vi "Find Config DB.vi"(8 "error in (no error)":errorcluster, 11 "Elevator Controller in":refnum<class "Elevator Controller.lvclass">) -> (0 "error out":errorcluster, 2 "DB Found?":bool, 3 "Elevator Controller out":refnum<class "Elevator Controller.lvclass">)   [LabVIEW 2019, in "Elevator Controller Actor.lvlib" / "Elevator Controller.lvclass"]
uses:
  Elevator Controller.lvclass
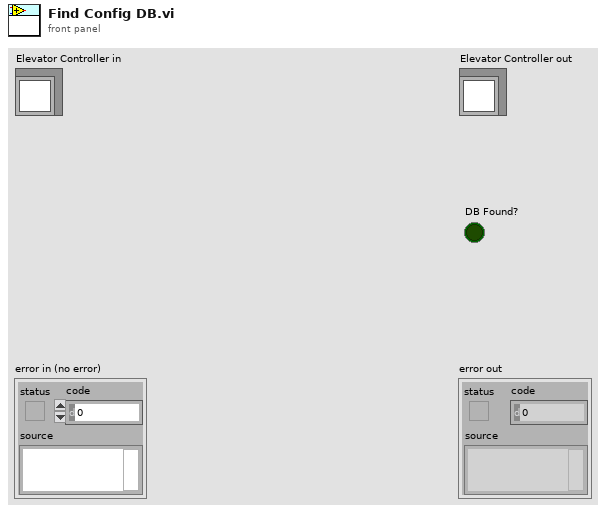
[diagram p1: front panel]
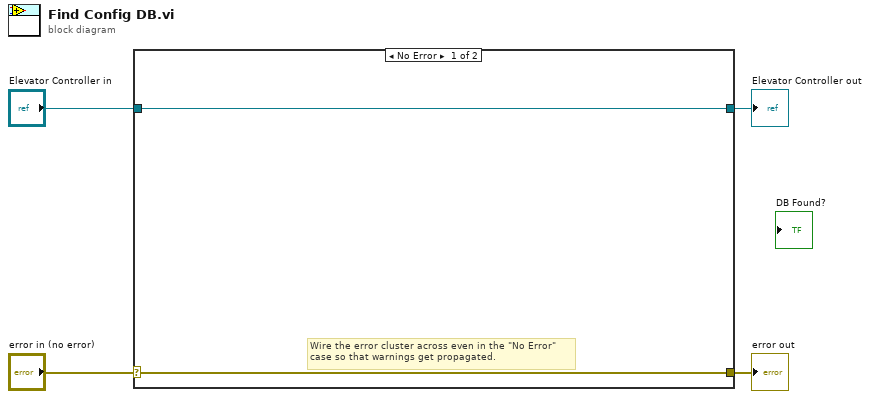
[diagram p0: block diagram]
diagram:
  n1 = case shown="No Error" "error in (no error)" {
    selector: "error in (no error)" -> [w5 w8]
    tunnel: [w5 w8] -> w3
    tunnel: [w6 w7] -> w1
    tunnel: "Elevator Controller in" -> [w6 w7]
    frame No Error {
      # "Wire the error cluster across even in the \"No Error\"\ncase so that warnings get propagated."
    }
    frame Error {
    }
  }
  "error out" <- w3
  "Elevator Controller out" <- w1
